vi "Resolve Mapped Path To Drive Letter.vi"(0 "Mapped Path":path, 11 "error in (no error)":errorcluster) -> (4 "Drive Letter":string, 6 "Found":bool, 15 "error out":errorcluster)   [LabVIEW 2017, in "G3_Build Process File Utilities.lvlib"]
uses:
  G3_Build Process File Utilities.lvlib
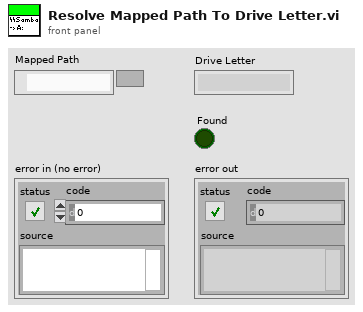
[diagram p1: front panel]
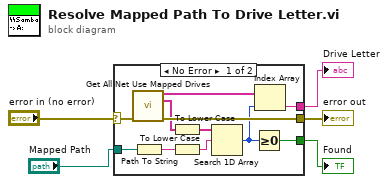
[diagram p0: block diagram]
diagram:
  n1 = case shown="No Error" "error in (no error)" {
    selector: "error in (no error)" -> [w14 w17]
    tunnel: "Mapped Path" -> [w16 _]
    tunnel: [w15 _] -> w4
    tunnel: [w13 w17] -> w2
    tunnel: [w7 _] -> w1
    frame No Error {
      n2 = call "Get All Net Use Mapped Drives.vi"("error in (no error)"=w14) -> ("Mapped Drive Letters"=w11:string[], "Mapped Paths"=w12:string[], "error out"=w13:errorcluster)  [unwired: 12 in]
      n3 = Path To String(path=w16) -> (string=w6:string)
      n4 = To Lower Case(string=w12) -> (all lower case string=w10:string[])
      n5 = To Lower Case(string=w6) -> (all lower case string=w9:string)
      n6 = Search 1D Array(1D array=w10, element=w9) -> (index of element=w8:i32)  [unwired: 1 in]
      n7 = Greater Or Equal To 0?(x=w8) -> (x >= 0?=w7:bool)
      n8 = Index Array(array=w11, index=w8) -> (element=w15:string)
    }
    frame Error {
    }
  }
  "Drive Letter" <- w4
  "error out" <- w2
  "Found" <- w1
